vi "PI dbToStr.vi"(6 "Axes":string=" A", 9 "Start":dbl, 10 "String in":string) -> (2 "String out":string)   [LabVIEW 2020]
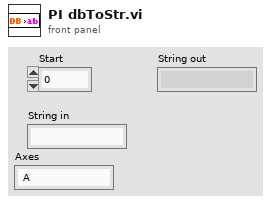
[diagram p1: front panel]
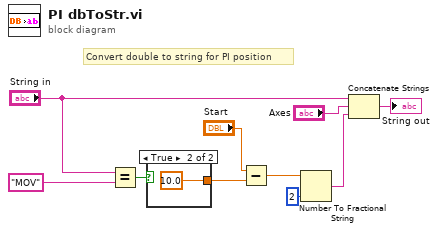
[diagram p0: block diagram]
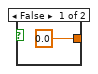
[diagram p2: hidden frame]
diagram:
  # "Convert double to string for PI position"
  n1 = Equal?(x="String in", y="MOV") -> (x = y?=w2:bool)
  n2 = case shown="True" w2 {
    tunnel: [0.0 ("y") 10.0 ("y")] -> w4
    frame False {
    }
    frame True {
    }
  }
  n3 = Subtract(x="Start", y=w4) -> (x-y=w6:dbl)
  n4 = Number To Fractional String(number=w6, precision (6)=i16 2) -> (F-format string=w8:string)  [unwired: 2 in]
  n5 = Concatenate Strings("String in", "Axes", w8) -> (→"String out":string)
